vi "TDC_DAQV_CountingRate.vi"(4 "Thresholds (mV)":u16[](array[numeric])=[580, 580, 580, 580, 600, 600, 600, 600, 580, 580, 600, 600, 600, 600, 600, 600, 580, 580, 600, 600, 600, 600, 600, 600, 580, 580, 600, 600, 600, 600, 600, 600], 5 "Thresholds":u16=590, 6 "address":string="192.168.10.22", 7 "bytes to read":i32=1600, 8 "error in (no error)":errorcluster, 9 "UDP Config":bool=TRUE, 10 "timeout":dbl=20.0, 11 "SMA mode":bool) -> (0 "error out":errorcluster={"status"=TRUE, "code"=56, "source"="TCP Read in TDC_DAQV_CountingRate.vi->baseline_scanV2.vi"}, 1 "rate_array":dbl[](array[numeric])=[163.0, 172.0, 236.0, 80.0, 68.0, 14.0, -1.0, -1.0, -1.0, -1.0, -1.0, 1033.0, -1.0, -1.0, -1.0, -1.0, 14959.0, 2904.0, 2688.0, 2241.0, 1909.0, 714.0, -1.0, -1.0, 775.0, 1180.0, 706.0, 10.0, 472.0, 672.0, -1.0, -1.0], 2 "time":dbl=3.2112889289855957, 3 "rate":dbl)   [LabVIEW 2017]
panel:
  out "rate_array 2":dbl[](array[numeric])=[163.0, 172.0, 236.0, 80.0, 68.0, 14.0, -1.0, -1.0, -1.0, -1.0, -1.0, 1033.0, -1.0, -1.0, -1.0, -1.0, 14959.0, 2904.0, 2688.0, 2241.0, 1909.0, 714.0, -1.0, -1.0, 775.0, 1180.0, 706.0, 10.0, 472.0, 672.0, -1.0, -1.0]
  out "数值":dbl
  out "sent number 2":u64=14726539 format="%x"
  out "data 9":string
  out "sent number":u64=224 format="%x"
  out "substring 2":string
  out "channel number":u64=4 format="%x"
  out "substring":string
  out "array":dbl[](array[numeric])=[-1.0, -1.0, -1.0, -1.0, -1.0, -1.0, -1.0, -1.0, -1.0, -1.0, -1.0, -1.0, -1.0, -1.0, -1.0, -1.0, -1.0, -1.0, -1.0, -1.0, -1.0, -1.0, -1.0, -1.0, -1.0, -1.0, -1.0, -1.0, -1.0, -1.0, -1.0, -1.0, -1.0, -1.0, -1.0, -1.0, -1.0, -1.0, -1.0, -1.0, -1.0, -1.0, -1.0, -1.0, -1.0, -1.0, -1.0, -1.0, -1.0, -1.0, -1.0, -1.0, -1.0, -1.0, -1.0, -1.0, -1.0, -1.0, -1.0, -1.0, -1.0, -1.0, -1.0, -1.0]
  out "trigger number":u64=46475 format="%x"
  out "data 8":string="祴"
  out "concatenated string":string
  out "number":u32=22
  in  "factor":i32=2
  in  "one key for threshold":bool=TRUE
  in  "stop":bool
  in  "timeout (ms)":i32=8400
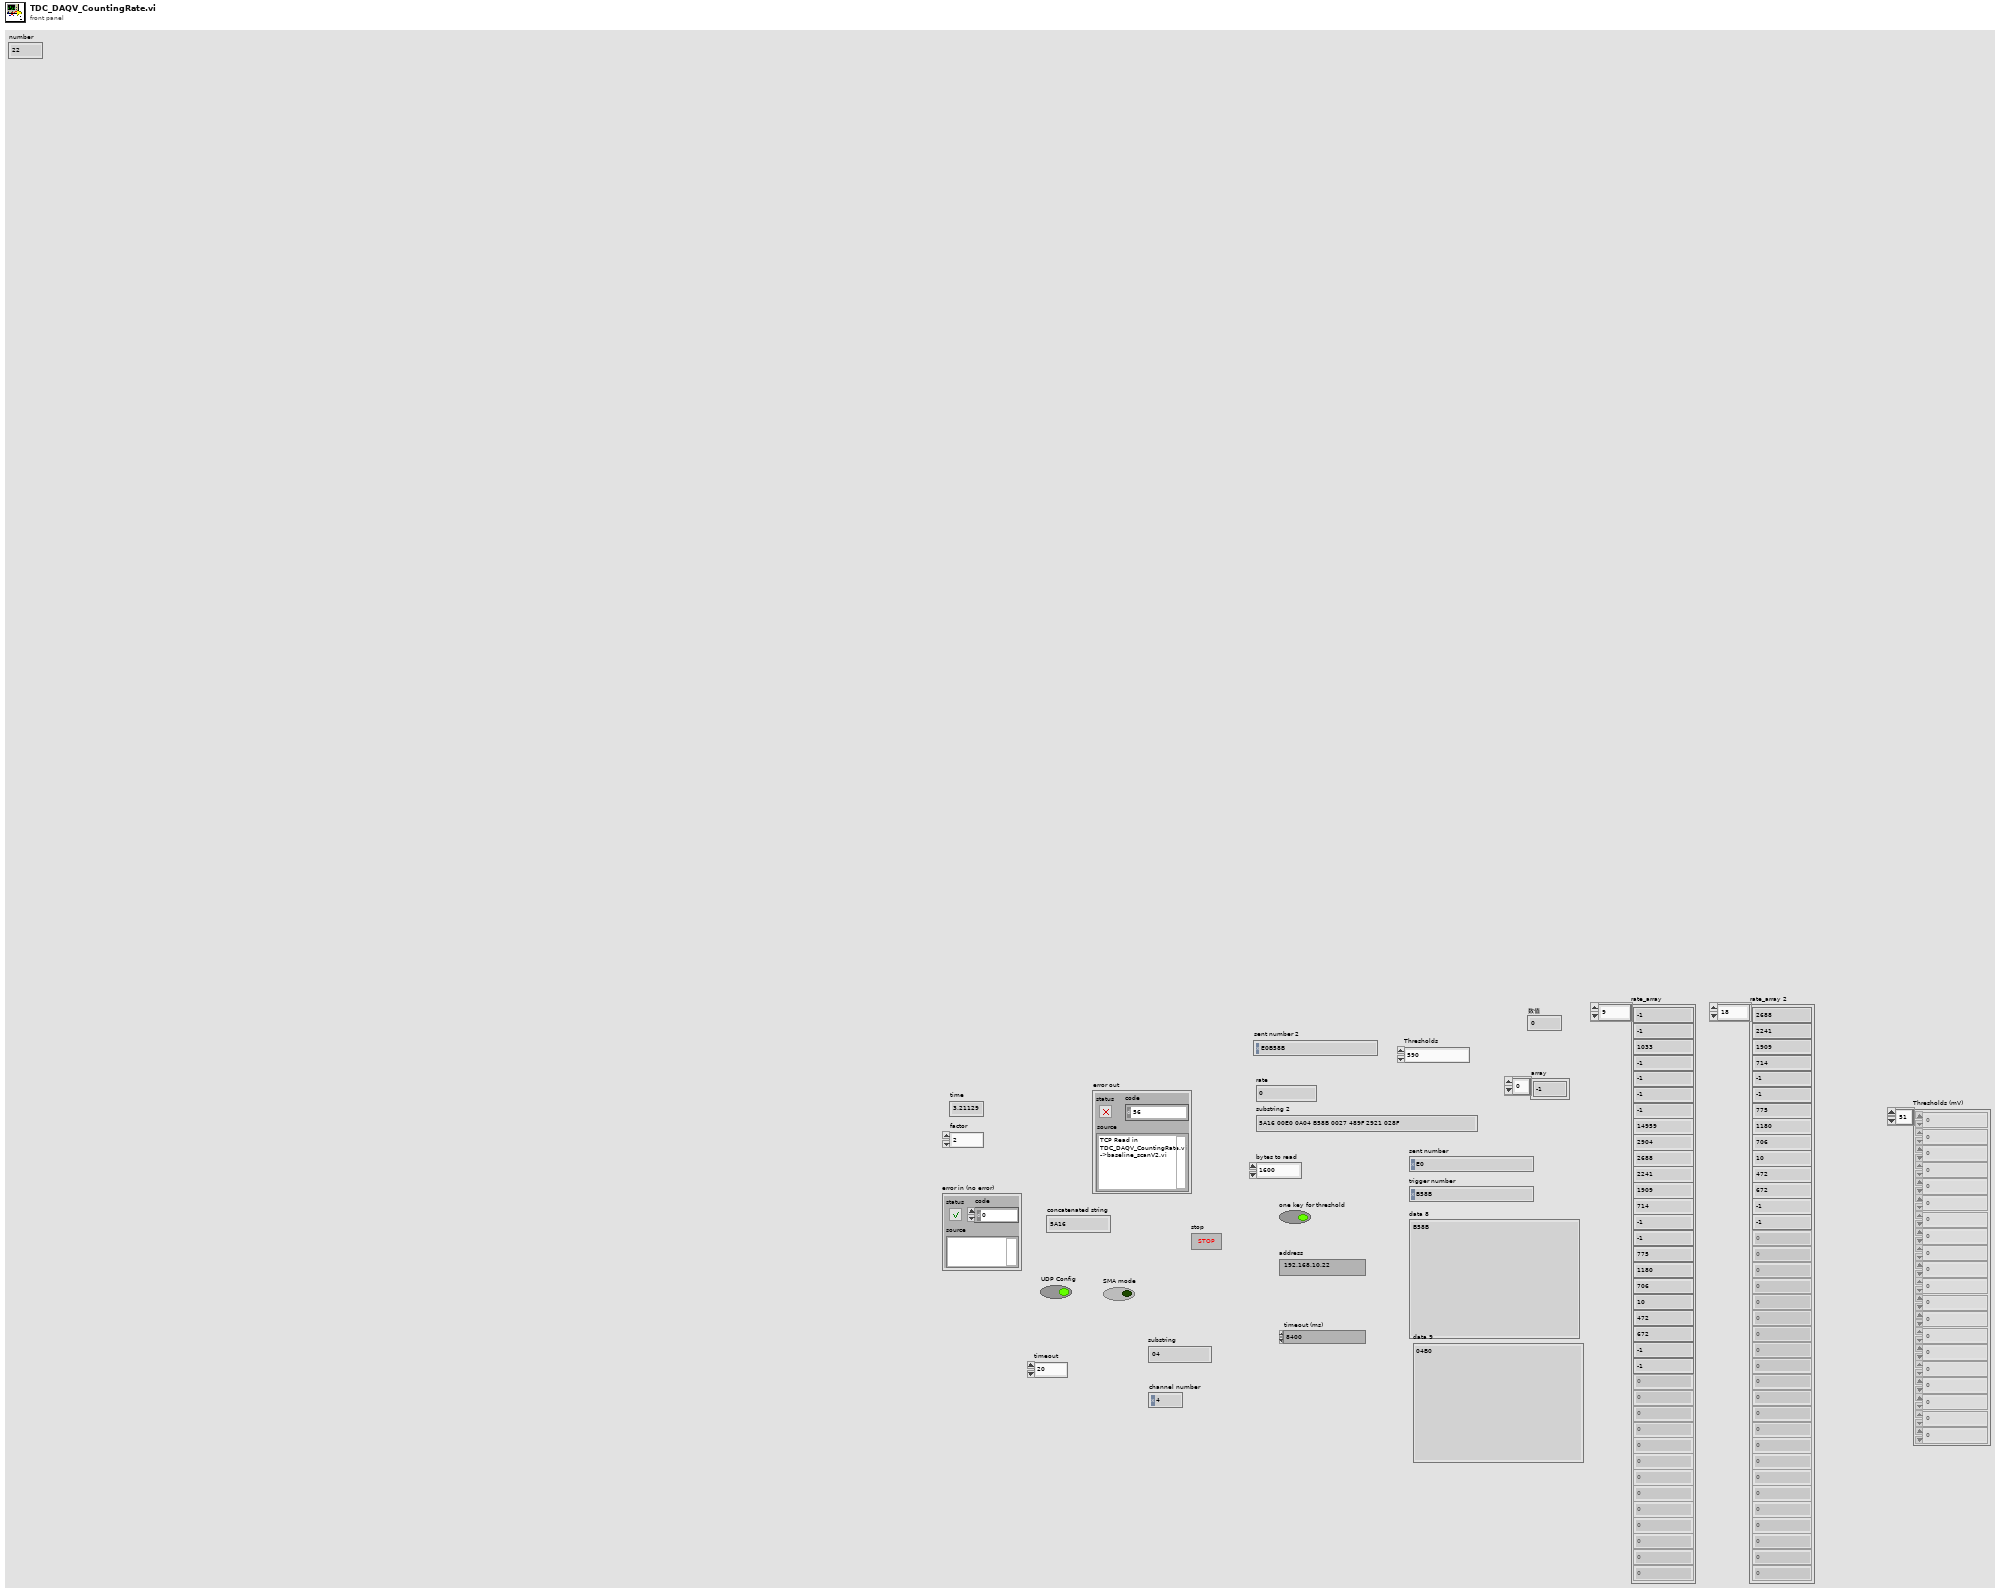
[diagram p1: front panel]
types:
  T1 = enum16{"Standard", "Buffered", "CRLF", "Immediate"}
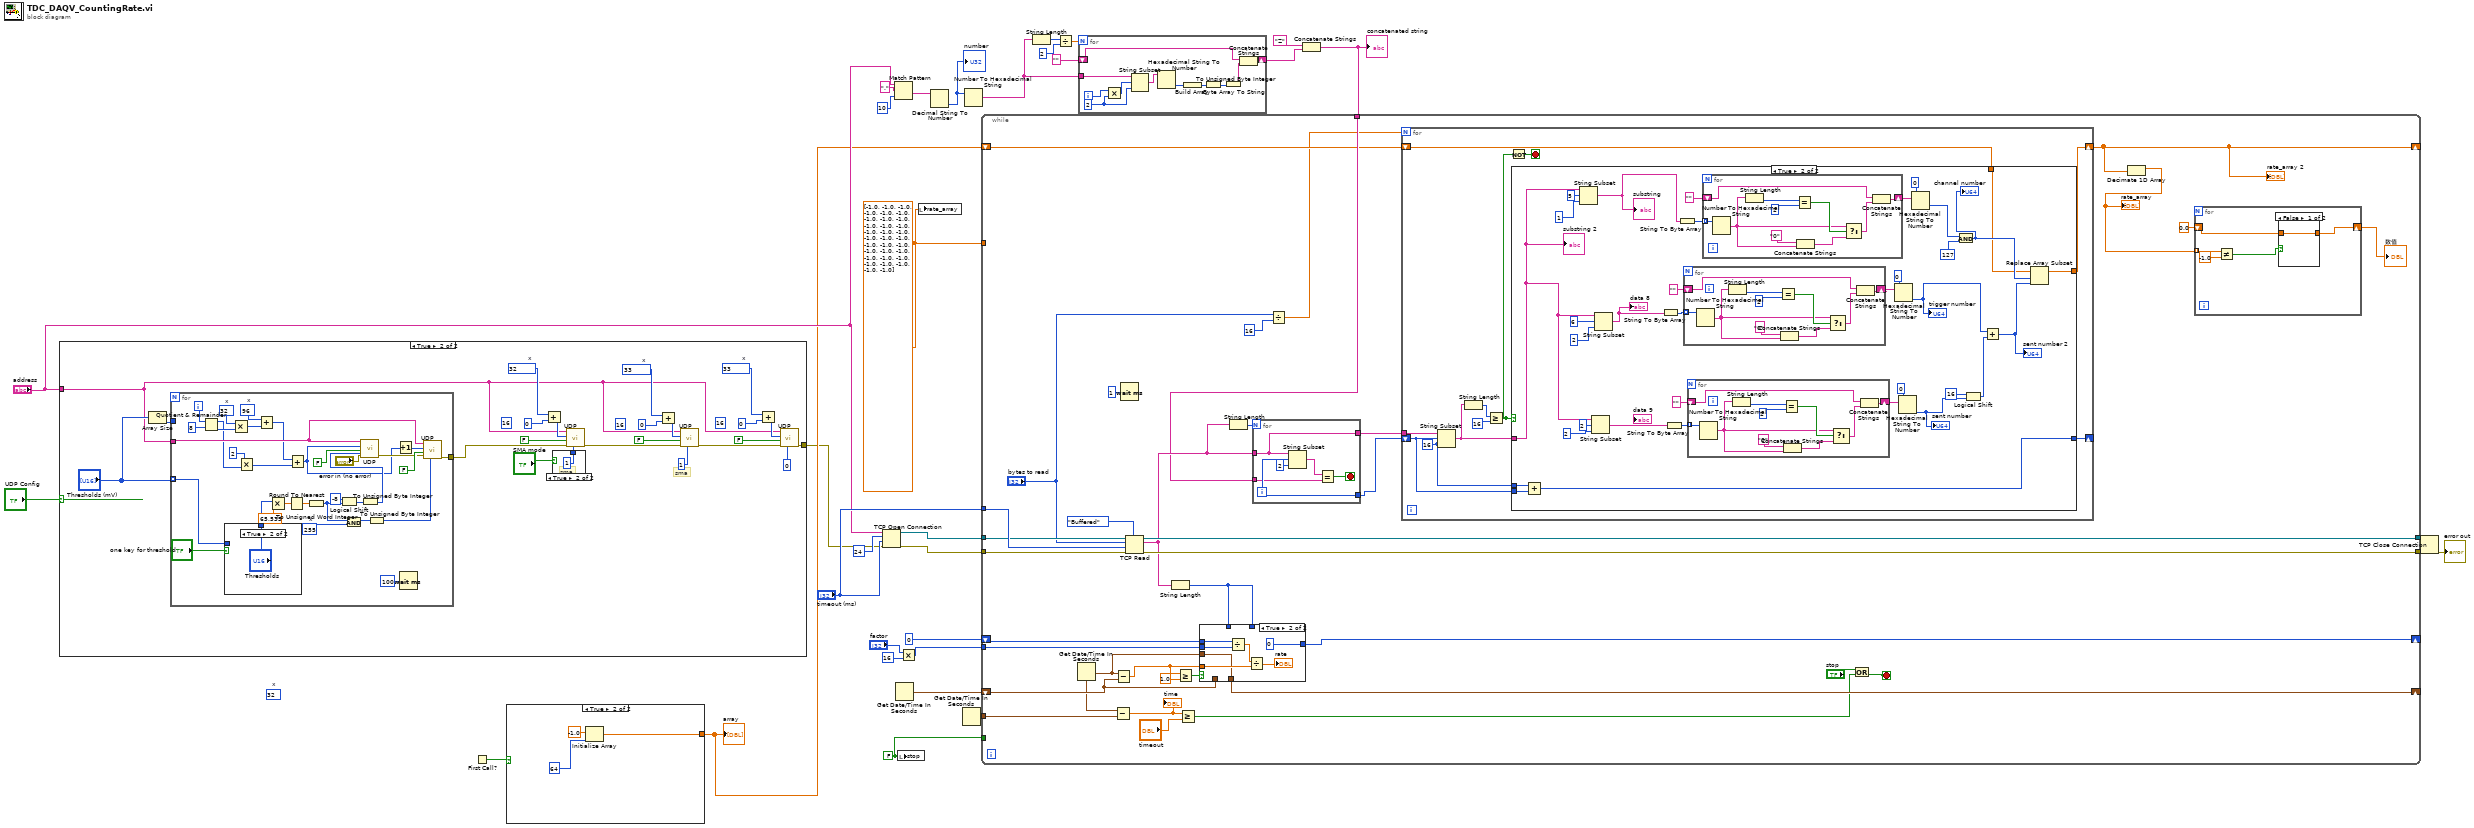
[diagram p0: block diagram]
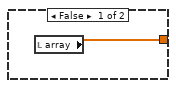
[diagram p2: hidden frame]
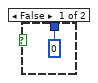
[diagram p4: hidden frame]
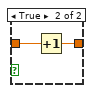
[diagram p6: hidden frame]
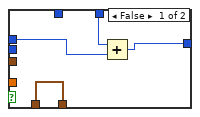
[diagram p8: hidden frame]
diagram:
  w1 = dbl[] [-1.0, -1.0, -1.0, -1.0, -1.0, -1.0, -1.0, -1.0, -1.0, -1.0, -1.0, -1.0, -1.0, -1.0, -1.0, -1.0, -1.0, -1.0, -1.0, -1.0, -1.0, -1.0, -1.0, -1.0, -1.0, -1.0, -1.0, -1.0, -1.0, -1.0, -1.0, -1.0] ("rate_array")
  w19 = FALSE ("stop")
  (unwired) u16 32  # x
  n1 = case shown="True" "UDP Config" {
    tunnel: "address" -> [_ w34]
    tunnel: [_ w33] -> w2
    frame False {
    }
    frame True {
      (unwired) u32 16 ("Address")
      w38 = u16 33  # x
      (unwired) u32 16 ("Address")
      w45 = u16 33  # x
      (unwired) u32 16 ("Address")
      w48 = u16 32  # x
      # "sma"
      n2 = Array Size(array="Thresholds (mV)") -> (size(s)=w51:i32)
      n3 = for {
        tunnel: w34 -> [w84]
        tunnel: "Thresholds (mV)" -> [w71] mode=indexing
        tunnel: [w74] -> w54
        tunnel: w51 -> [_]
        i -> [w66]
        w67 = u16 96  # x
        w68 = u16 32  # x
        w80 = u16 255  # x
        n4 = Quotient & Remainder(x=w66, y=8) -> (x-y*floor(x/y)=w60:i32, floor(x/y)=w69:i32)
        n5 = case shown="True" "one key for threshold" {
          tunnel: [w90 "Thresholds"] -> w72
          tunnel: w71 -> [w90 _]
          frame False {
          }
          frame True {
          }
        }
        n6 = Multiply(x=w68, y=w69) -> (x*y=w63:i32)
        n7 = Multiply(x=2, y=w60) -> (x*y=w61:i32)
        n8 = Add(x=w67, y=w63) -> (x+y=w62:i32)
        n9 = Multiply(x=w72, y=65.535) -> (x*y=w87:dbl)
        n10 = Round To Nearest(number=w87) -> (nearest integer value=w85:dbl)
        n11 = Add(x=w62, y=w61) -> (x+y=w65:i32)
        n12 = To Unsigned Word Integer(number=w85) -> (unsigned 16bit integer=w76:u16)
        n13 = Logical Shift(y=i16 -8, x=w76) -> (x << y=w82:u16)
        n14 = And(x=w76, y=w80) -> (x .and. y?=w79:u16)
        n15 = To Unsigned Byte Integer(number=w82) -> (unsigned 8bit integer=w81:u8)
        n16 = call "UDP.vi"("In"=w81, "error in (no error)"="error in (no error)", "Read (TRUE)"=FALSE, "Address"=w65, "IP address"=w84) -> ("error out"=w75:errorcluster)  [unwired: 3 in, 2 out]
        n17 = To Unsigned Byte Integer(number=w79) -> (unsigned 8bit integer=w78:u8)
        n18 = Increment(x=w65) -> (x+1=w64:i32)
        n19 = Wait (ms)(milliseconds to wait=u32 100) -> ()  [unwired: 1 out]
        n20 = call "UDP.vi"("In"=w78, "error in (no error)"=w75, "Read (TRUE)"=FALSE, "Address"=w64, "IP address"=w84) -> ("error out"=w74:errorcluster)  [unwired: 3 in, 2 out]
      }
      n21 = Add(x=w48, y=u32 0 ("Address")) -> (x+y=w47:u32)
      n22 = case shown="True" "SMA mode" {
        tunnel: [u8 0 ("In") u8 1 ("In")] -> w53
        frame False {
        }
        frame True {
          # "sma"
        }
      }
      n23 = call "UDP.vi"("In"=w53, "error in (no error)"=w54, "Read (TRUE)"=FALSE, "Address"=w47, "IP address"=w34) -> ("error out"=w36:errorcluster)  [unwired: 3 in, 2 out]
      n24 = Add(x=w45, y=u32 0 ("Address")) -> (x+y=w46:u32)
      n25 = call "UDP.vi"("In"=u8 1, "error in (no error)"=w36, "Read (TRUE)"=FALSE, "Address"=w46, "IP address"=w34) -> ("error out"=w35:errorcluster)  [unwired: 3 in, 2 out]
      n26 = Add(x=w38, y=u32 0 ("Address")) -> (x+y=w37:u32)
      n27 = call "UDP.vi"("In"=u8 0, "error in (no error)"=w35, "Read (TRUE)"=FALSE, "Address"=w37, "IP address"=w34) -> ("error out"=w33:errorcluster)  [unwired: 3 in, 2 out]
    }
  }
  n28 = First Call?() -> (First Call?: T/F=w4:bool)
  n29 = case shown="True" w4 {
    tunnel: [w92 w93] -> w3
    frame False {
      n30 = local read "array"() -> (w92:dbl[])
    }
    frame True {
      n31 = Initialize Array(-1.0 ("element"), 64 ("dimension size")) -> (w93:dbl[])
    }
  }
  "array" <- w3
  n32 = TCP Open Connection(address="address", remote port or service name=u16 24 ("port"), timeout ms (60000)="timeout (ms)", error in (no error)=w2) -> (connection ID=w30:refnum<k5>, error out=w31:errorcluster)  [unwired: 1 in]
  n33 = Match Pattern(string="address", regular expression="." ("search string"), offset (0)=10) -> (after substring=w10:string)  [unwired: 3 out]
  n34 = Get Date/Time In Seconds() -> (seconds since 1Jan1904=w25:timestamp)
  n35 = local write "stop"(w19) -> ()
  n36 = Multiply(x="factor", y=16) -> (x*y=w21:i32)
  n37 = local write "rate_array"(w1) -> ()
  n38 = Decimal String To Number(string=w10) -> (number=w9:i32)  [unwired: 2 in, 1 out]
  "number" <- w9
  n39 = Get Date/Time In Seconds() -> (seconds since 1Jan1904=w18:timestamp)
  n40 = Number To Hexadecimal String(2:w9) -> (0:w8:string)  [unwired: 1 in]
  n41 = String Length(string=w8) -> (length=w15:i32)
  n42 = Divide(x=w15, y=2) -> (x/y=w16:dbl)
  n43 = for {
    N: w16 -> [_]
    shift-right: [w106] -> w7
    shift-left: "" ("format string") -> [w105]
    tunnel: w8 -> [w96]
    i -> [w104]
    w98 = 2 ("y")
    n44 = Multiply(x=w104, y=w98) -> (x*y=w97:i32)
    n45 = String Subset(string=w96, offset (0)=w97, length (rest)=w98) -> (substring=w99:string)
    n46 = Hexadecimal String To Number(string=w99) -> (number=w103:u32)  [unwired: 2 in, 1 out]
    n47 = Build Array(w103) -> (w102:u32[])
    n48 = To Unsigned Byte Integer(number=w102) -> (unsigned 8bit integer=w101:u8[])
    n49 = Byte Array To String(unsigned byte array=w101) -> (string=w100:string)
    n50 = Concatenate Strings(w105, w100) -> (w106:string)
  }
  n51 = Concatenate Strings("Z", w7) -> (w5:string)
  "concatenated string" <- w5
  n52 = while {
    tunnel: w31 -> [w142]
    tunnel: "timeout (ms)" -> [w141]
    tunnel: w30 -> [w140]
    tunnel: [w139] -> w29
    tunnel: [w138] -> w28
    shift-right: [w131] -> _
    shift-left: w25 -> [w135]
    shift-right: [w134] -> _
    shift-left: u32 0 ("milliseconds to wait") -> [w129]
    tunnel: w21 -> [w128]
    tunnel: w19 -> [_]
    tunnel: w18 -> [w122]
    tunnel: w5 -> [w116]
    shift-right: [w107] -> _
    shift-left: w3 -> [w115]
    tunnel: w1 -> [_]
    stop <- w125 stop-if-true
    n53 = Get Date/Time In Seconds() -> (seconds since 1Jan1904=w121:timestamp)
    n54 = Subtract(x=w121, y=w122) -> (x-y=w120:dbl)
    "time" <- w120
    n55 = Subtract(x=w121, y=w135) -> (x-y=w127:dbl)
    n56 = Wait (ms)(milliseconds to wait=u32 1) -> ()  [unwired: 1 out]
    n57 = TCP Read(connection ID=w140, bytes to read="bytes to read", error in (no error)=w142, 7:T1."Buffered" ("mode (standard)"), 9:w141) -> (connection ID out=w139:refnum<k5>, data out=w117:string, error out=w138:errorcluster)
    n58 = String Length(string=w117) -> (length=w130:i32)
    n59 = Greater Or Equal?(x=w127, y=1.0) -> (x >= y?=w133:bool)
    n60 = Greater Or Equal?(x=w120, y="timeout") -> (x >= y?=w123:bool)
    n61 = case shown="True" w133 {
      tunnel: w127 -> [_ w245]
      tunnel: w121 -> [_ w243]
      tunnel: [w238 w243] -> w131
      tunnel: w135 -> [w238 _]
      tunnel: w130 -> [_ _]
      tunnel: w130 -> [w237 _]
      tunnel: [w236 0] -> w134
      tunnel: w128 -> [_ w240]
      tunnel: w129 -> [w235 w239]
      frame False {
        n62 = Add(x=w237, y=w235) -> (x+y=w236:u32)
      }
      frame True {
        n63 = Divide(x=w239, y=w240) -> (x/y=w242:dbl)
        n64 = Divide(x=w242, y=w245) -> (x/y=→"rate":dbl)
      }
    }
    n65 = String Length(string=w117) -> (length=w119:i32)
    n66 = for {
      N: w119 -> [_]
      tunnel: w117 -> [w231]
      tunnel: [w231] -> w118
      tunnel: [w230] -> w114
      tunnel: w116 -> [w229]
      i -> [w230]
      stop <- w232 stop-if-true
      n67 = String Subset(string=w231, offset (0)=w230, length (rest)=2 ("length (rest)")) -> (substring=w233:string)
      n68 = Equal?(x=w233, y=w229) -> (x = y?=w232:bool)
    }
    n69 = Divide(x="bytes to read", y=16 ("length (rest)")) -> (x/y=w111:dbl)
    n70 = for {
      N: w111 -> [_]
      tunnel: w118 -> [w161]
      shift-right: [w159] -> w107
      shift-left: w115 -> [w160]
      shift-right: [w151] -> _
      shift-left: w114 -> [w152]
      stop <- w154 stop-if-true
      w153 = 16 ("length (rest)")
      n71 = String Subset(string=w161, offset (0)=w152, length (rest)=w153) -> (substring=w158:string)
      n72 = String Length(string=w158) -> (length=w157:i32)
      n73 = Greater Or Equal?(x=w157, y=16 ("length (rest)")) -> (x >= y?=w155:bool)
      n74 = Not(x=w155) -> (.not. x?=w154:bool)
      n75 = case shown="True" w155 {
        tunnel: w158 -> [_ w179]
        tunnel: w160 -> [w163 w178]
        tunnel: [w163 w177] -> w159
        tunnel: w152 -> [w162 w176]
        tunnel: w153 -> [_ w175]
        tunnel: [w162 w174] -> w151
        frame False {
        }
        frame True {
          n76 = Add(x=w175, y=w176) -> (x+y=w174:i32)
          n77 = String Subset(string=w179, offset (0)=5, length (rest)=1 ("length (rest)")) -> (substring=w183:string)
          "substring" <- w183
          n78 = String Subset(string=w179, offset (0)=2, length (rest)=2 ("length (rest)")) -> (substring=w169:string)
          n79 = String Subset(string=w179, offset (0)=6, length (rest)=2 ("length (rest)")) -> (substring=w190:string)
          "data 8" <- w190
          n80 = String To Byte Array(string=w190) -> (unsigned byte array=w192:u8[])
          n81 = String To Byte Array(string=w169) -> (unsigned byte array=w172:u8[])
          n82 = String To Byte Array(string=w183) -> (unsigned byte array=w186:u8[])
          n83 = for {
            shift-right: [w227] -> w193
            shift-left: "" ("format string") -> [w224]
            tunnel: w192 -> [w228] mode=indexing
            n84 = Number To Hexadecimal String(2:w228) -> (0:w220:string)  [unwired: 1 in]
            n85 = String Length(string=w220) -> (length=w226:i32)
            n86 = Equal?(x=w226, y=2) -> (x = y?=w223:bool)
            n87 = Concatenate Strings("0" ("format string"), w220) -> (w222:string)
            n88 = Select(t=w220, s=w223, f=w222) -> (s? t:f=w219:string)
            n89 = Concatenate Strings(w224, w219) -> (w227:string)
          }
          n90 = for {
            shift-right: [w207] -> w171
            shift-left: "" ("format string") -> [w204]
            tunnel: w172 -> [w208] mode=indexing
            n91 = Number To Hexadecimal String(2:w208) -> (0:w200:string)  [unwired: 1 in]
            n92 = String Length(string=w200) -> (length=w206:i32)
            n93 = Equal?(x=w206, y=2) -> (x = y?=w203:bool)
            n94 = Concatenate Strings("0" ("format string"), w200) -> (w202:string)
            n95 = Select(t=w200, s=w203, f=w202) -> (s? t:f=w199:string)
            n96 = Concatenate Strings(w204, w199) -> (w207:string)
          }
          n97 = for {
            shift-right: [w217] -> w185
            shift-left: "" ("format string") -> [w214]
            tunnel: w186 -> [w218] mode=indexing
            n98 = Number To Hexadecimal String(2:w218) -> (0:w210:string)  [unwired: 1 in]
            n99 = String Length(string=w210) -> (length=w216:i32)
            n100 = Equal?(x=w216, y=2) -> (x = y?=w213:bool)
            n101 = Concatenate Strings("0" ("format string"), w210) -> (w212:string)
            n102 = Select(t=w210, s=w213, f=w212) -> (s? t:f=w209:string)
            n103 = Concatenate Strings(w214, w209) -> (w217:string)
          }
          n104 = Hexadecimal String To Number(string=w193, default (0uL)=u64 0 ("default (0 U32)")) -> (number=w166:u64)  [unwired: 1 in, 1 out]
          "trigger number" <- w166
          n105 = Hexadecimal String To Number(string=w171, default (0uL)=u64 0 ("default (0 U32)")) -> (number=w168:u64)  [unwired: 1 in, 1 out]
          "sent number" <- w168
          n106 = Hexadecimal String To Number(string=w185, default (0uL)=u64 0 ("default (0 U32)")) -> (number=w182:u64)  [unwired: 1 in, 1 out]
          n107 = And(x=w182, y=u64 127 ("default (0 U32)")) -> (x .and. y?=w180:u64)
          "channel number" <- w180
          n108 = Logical Shift(y=i16 16, x=w168) -> (x << y=w165:u64)
          n109 = Add(x=w166, y=w165) -> (x+y=w164:u64)
          "sent number 2" <- w164
          n110 = Replace Array Subset(array=w178, new element=w164, index=w180) -> (w177:dbl[])
          "substring 2" <- w179
        }
      }
    }
    "rate_array 2" <- w107
    n111 = Or(x="stop", y=w123) -> (x .or. y?=w125:bool)
    n112 = Decimate 1D Array(w107) -> (w110:dbl[])  [unwired: 1 out]
    "rate_array" <- w110
    n113 = for {
      tunnel: w110 -> [w147] mode=indexing
      shift-right: [w143] -> w108
      shift-left: 0.0 -> [w144]
      n114 = Not Equal?(x=w147, y=-1.0) -> (x != y?=w145:bool)
      n115 = case shown="False" w145 {
        tunnel: w144 -> [w148 w150]
        tunnel: [w148 w149] -> w143
        frame False {
        }
        frame True {
          n116 = Increment(x=w150) -> (x+1=w149:dbl)
        }
      }
    }
    "数值" <- w108
  }
  n117 = TCP Close Connection(connection ID=w29, error in (no error)=w28) -> (error out=→"error out":errorcluster)  [unwired: 1 in, 1 out]
